vi "PH_Beckhoff-16BB.write Chiller to PSDB.vi"(0 "i ref in":refnum<vi>, 5 "error IO":errorcluster) -> (14 "i ref out":refnum<vi>, 19 "error out":errorcluster)   [LabVIEW 2014, in "PH_Beckhoff-16BB.lvlib"]
doc: "This VI writes the chiller data to the PHELIX shot data base."
uses:
  PH_Beckhoff-16BB.lvlib
  PH_StatusHandler/PH_StatusHandler.Status.ctl
  PH_PSDBWriter/PH_PSDBWriter.Data Status.ctl
  PH_Beckhoff/PH_Beckhoff.lvlib
  CSCore/CSSystem/CSSystemLib/CSSystemLib.lvlib
  PH_PSDBWriter/PH_PSDBWriter.lvlib
  PH_Common/PH_Common.lvlib
  PH_StatusHandler/PH_StatusHandler.lvlib
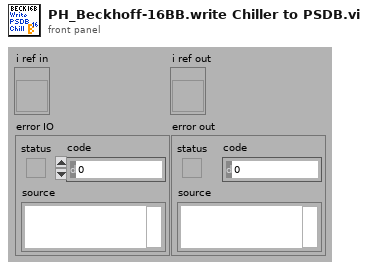
[diagram p1: front panel]
types:
  T1 = typedef "PH_Beckhoff.lvlib/PH_Beckhoff.i attribute.ctl" = cluster{"GUI Refs":T2, "operation?":bool, "Default Prdc Interval":i32, "Connection":T3, "AMS Net ID":T4, "Klemmencluster: # of":T5, "Values":T6, "IP":string, "Description":string, "configured?":bool, "Change Manager":cluster{"Detemination wanted?":bool, "Values changed at":cluster{"Sonderklemmen Inputs":i32[], "Analog Inputs":i32[], "Analog Outputs":i32[], "Digital Inputs":i32[], "Digital Outputs":i32[]}}, "Difference to handle an analog input as change":u32}
  T2 = typedef "PH_Beckhoff.lvlib/PH_Beckhoff.GUI Refs.ctl" = cluster{"ADS Error":refnum<vi>, "Values":refnum<vi>, "configured?":refnum<vi>, "Connection":refnum<vi>, "IP":refnum<vi>, "Prdc Int [ms]":refnum<vi>}
  T3 = typedef "PH_Beckhoff.lvlib/PH_Beckhoff.Connectivity.ctl" = cluster{"DLL?":bool, "Port?":bool, "Client?":bool, "Ping?":bool, "unsuccessful Pings":u32}
  T4 = typedef "Beckhoff - Driver np.lvlib/Beckhoff Access.ctl" = cluster{"DLL path":path, "AMS Net ID":cluster{"1st # of IP":u8, "2nd # of IP":u8, "3rd # of IP":u8, "4th # of IP":u8, "In Port":u8, "Out Port":u8}}
  T5 = typedef "Beckhoff - Driver np.lvlib/Klemmendeclarer.ctl" = cluster{"Offset due to Sonderklemms":u32, "analog Inputs":u32, "analog Outputs":u32, "digital Input Bits":u32, "digital Output Bits":u32}
  T6 = typedef "PH_Beckhoff.lvlib/PH_Beckhoff.Values.ctl" = cluster{"Sonderklemmen Inputs":T7, "Analog Inputs":T8, "Analog Outputs":T10, "Digital Inputs":T11, "Digital Outputs":T12}
  T7 = typedef "PH_Beckhoff.lvlib/PH_Beckhoff.Sonderklemmen Inputs.ctl" = cluster{"Total Length":u32, "Name":string, "Value":u64, "Quality":bool, "Service ID":i32, "Offset":u32, "Length":u32}[]
  T8 = typedef "PH_Beckhoff.lvlib/PH_Beckhoff.Analog Inputs.ctl" = cluster{"Name":string, "Value":u32, "Quality":bool, "Service ID":i32, "Sca Type":T9}[]
  T9 = typedef "PH_Beckhoff.lvlib/PH_Beckhoff.Scaling Type.ctl" = enum16{"none", "0 ... 15 Bit -> 0 ... 5", "0 ... 15 Bit -> 0 ... 10", "0 ... 15 Bit -> 0 ... 25", "0 ... 15 Bit -> 4 ... 20", "0 ... 15 Bit -> 0 ... 1", "0 ... 15 Bit -> 0 ... 20000", "0 ... 15 Bit -> 0 ... 24000"}
  T10 = typedef "PH_Beckhoff.lvlib/PH_Beckhoff.Analog Outputs.ctl" = cluster{"Name":string, "Value":u32, "Quality":bool, "Wanted Value":u32, "Service ID":i32, "Sca Type":T9}[]
  T11 = typedef "PH_Beckhoff.lvlib/PH_Beckhoff.Digital Inputs.ctl" = cluster{"Name":string, "Value":bool, "Quality":bool, "Service ID":i32, "inverted?":bool}[]
  T12 = typedef "PH_Beckhoff.lvlib/PH_Beckhoff.Digital Outputs.ctl" = cluster{"Name":string, "Value":bool, "Quality":bool, "Wanted Value":bool, "Service ID":i32, "inverted?":bool}[]
  T13 = typedef "PH_Beckhoff-16BB.lvlib/PH_Beckhoff-16BB.i attribute.ctl" = cluster{"PA Chiller":cluster{"PSDB":cluster{"Status Service ID":i32, "Instance ID":i32, "Data Status":T14, "Ref Status":refnum<vi>, "Error Code":i32}, "Status":cluster{"GUI Ref":refnum<vi>, "Status Service ID":i32, "Status":T15}, "DIs":cluster{"Flow Control":cluster{"GUI Ref":refnum<vi>, "# in Data":i32}, "High-Temp":cluster{"GUI Ref":refnum<vi>, "# in Data":i32}, "Conductivity":cluster{"GUI Ref":refnum<vi>, "# in Data":i32}, "Niveau":cluster{"GUI Ref":refnum<vi>, "# in Data":i32}}, "PSDB Thread":cluster{"Ref":refnum<vi>, "Q-Ref":refnum<queue>}}, "PSDB":cluster{"Shot #":i32, "Subsystem":T16}, "Racktype":string, "PSDB Credentials":T17}
  T14 = typedef "PH_PSDBWriter.lvlib/PH_PSDBWriter.Data Status.ctl" = i16
  T15 = typedef "PH_StatusHandler.lvlib/PH_StatusHandler.Status.ctl" = i16
  T16 = typedef "PH_PSDBWriter.lvlib/PH_PSDBWriter.PHELIX-Subsystems.ctl" = i32
  T17 = typedef "PH_Common.lvlib/PH_Connection.PSDB Credentials.ctl" = cluster{"PW":string, "ID":string, "DS":string}
  T18 = typedef "PH_PSDBWriter.lvlib/PH_PSDBWriter.String dataset.ctl" = cluster{"name":string, "data":string, "unit":string}
  T19 = typedef "PH_PSDBWriter.lvlib/PH_PSDBWriter.PSDB Dataset.ctl" = cluster{"Version":i32, "2D data Input":T20[], "Boolean Input":T22[], "Image Input":T23[], "Numeric Input":T25[], "String Input":T18[]}
  T20 = typedef "PH_PSDBWriter.lvlib/PH_PSDBWriter.2D dataset.ctl" = cluster{"name":string, "data":dbl[][], "axis description":T21}
  T21 = typedef "PSDB.lvlib/PSDB_AxisDescription.ctl" = cluster{"x axis label":string, "y axis label":string, "x axis unit":string, "y axis unit":string}
  T22 = typedef "PH_PSDBWriter.lvlib/PH_PSDBWriter.Boolean dataset.ctl" = cluster{"name":string, "data":bool, "unit":string}
  T23 = typedef "PH_PSDBWriter.lvlib/PH_PSDBWriter.Image dataset.ctl" = cluster{"name":string, "data":T24, "unit":string}
  T24 = typedef "IMAQ Image.ctl" = refnum<image>
  T25 = typedef "PH_PSDBWriter.lvlib/PH_PSDBWriter.Numeric dataset.ctl" = cluster{"name":string, "data":dbl, "unit":string}
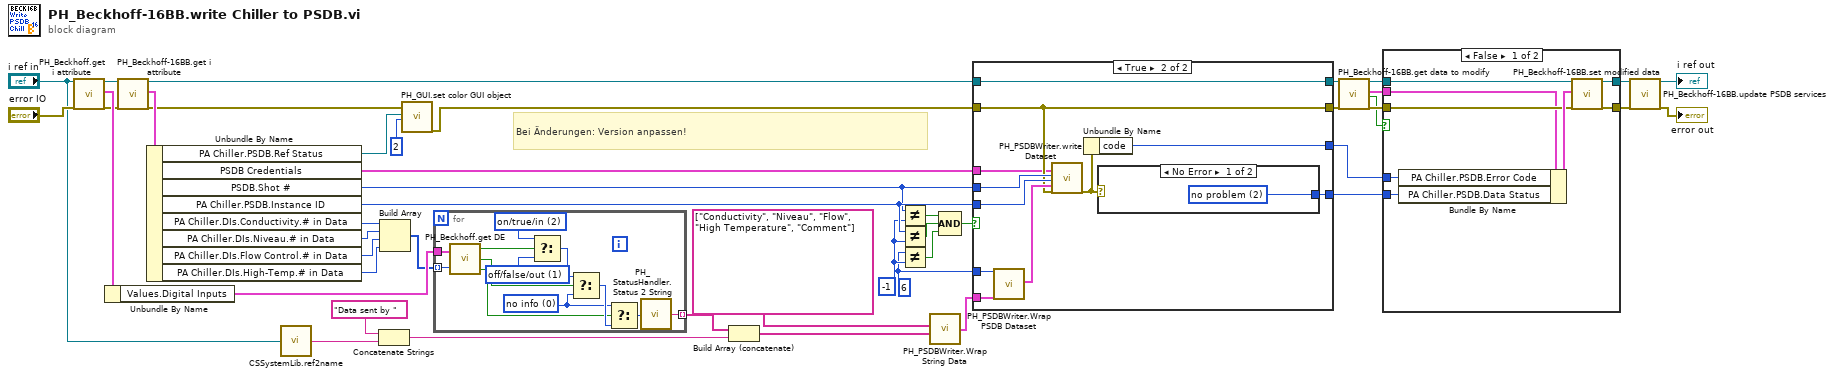
[diagram p0: block diagram]
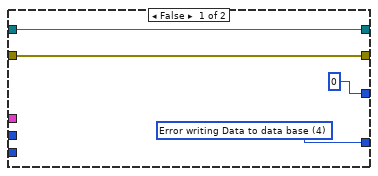
[diagram p3: hidden frame]
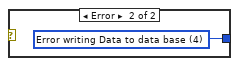
[diagram p4: hidden frame]
diagram:
  w34 = 6 ("Version")
  w40 = -1 ("y")
  # "Bei Änderungen: Version anpassen!"
  n1 = call "PH_Beckhoff.get i attribute.vi"("i ref in"="i ref in", "error in (no error)"="error IO") -> ("i ref out"=w12:refnum<vi>, "i attribute"=w23:T1, "error out"=w10:errorcluster)  [unwired: 15 in]
  n2 = Unbundle By Name(w23) -> ("Values.Digital Inputs"=w29:T11)
  n3 = call "PH_Beckhoff-16BB.get i attribute.vi"("i ref in"=w12, "error in (no error)"=w10) -> ("i ref out"=w11:refnum<vi>, "i attribute"=w9:T13, "error out"=w6:errorcluster)  [unwired: 15 in]
  n4 = Unbundle By Name(w9) -> ("PA Chiller.PSDB.Ref Status"=w8:refnum<vi>, "PSDB Credentials"=w1:T17, "PSDB.Shot #"=w42:i32, "PA Chiller.PSDB.Instance ID"=w43:i32, "PA Chiller.DIs.Conductivity.# in Data"=w33:i32, "PA Chiller.DIs.Niveau.# in Data"=w32:i32, "PA Chiller.DIs.Flow Control.# in Data"=w31:i32, "PA Chiller.DIs.High-Temp.# in Data"=w30:i32)
  n5 = call "CSSystemLib.ref2name.vi"("obj refnum"="i ref in") -> ("name"=w24:string)
  n6 = Concatenate Strings("Data sent by " ("string"), w24) -> (w25:string)
  n7 = Build Array(w33, w32, w31, w30) -> (w28:i32[])
  n8 = call "PH_GUI.set color GUI object.vi"("GUI object Ref"=w8, "State"=2, "error in (no error)"=w6) -> ("error out"=w5:errorcluster)  [unwired: 16 in]
  n9 = for {
    tunnel: [w51] -> w27 mode=indexing
    tunnel: w29 -> [w47]
    tunnel: w28 -> [w46] mode=indexing
    w53 = T15 1 items=["no info", "off/false/out", "on/true/in", "Failure", "Alarm", "Status 1", "Status 2", "Status 3"] ("State Temp not 2 low")
    w54 = T15 2 items=["no info", "off/false/out", "on/true/in", "Failure", "Alarm", "Status 1", "Status 2", "Status 3"] ("State Temp not 2 low")
    w56 = T15 0 items=["no info", "off/false/out", "on/true/in", "Failure", "Alarm", "Status 1", "Status 2", "Status 3"] ("State Temp not 2 low")
    n10 = call "PH_Beckhoff.get DE.vi"("Digital Values"=w47, "index of element"=w46) -> ("Value"=w50:bool, "Quality"=w49:bool, "Tag not found"=w48:bool)
    n11 = Select(t=w54, s=w50, f=w53) -> (s? t:f=w55:T15)
    n12 = Select(t=w55, s=w49, f=w56) -> (s? t:f=w57:T15)
    n13 = Select(t=w56, s=w48, f=w57) -> (s? t:f=w52:T15)
    n14 = call "PH_StatusHandler.Status 2 String.vi"("Status"=w52) -> ("Status as string"=w51:string)
  }
  n15 = Build Array (concatenate)(w27, w25) -> (w4:string[])
  n16 = Not Equal?(x=w42, y=w40) -> (x != y?=w39:bool)
  n17 = Not Equal?(x=w43, y=w40) -> (x != y?=w38:bool)
  n18 = Not Equal?(x=w34, y=w40) -> (x != y?=w37:bool)
  n19 = call "PH_PSDBWriter.Wrap String Data.vi"("Data Array"=w4, "Name Array"=string[] ["Conductivity", "Niveau", "Flow", "High Temperature", "Comment"]) -> ("PSDB String Data Array"=w2:T18[])  [unwired: 2 in]
  n20 = Compound Arithmetic op=AND(w39, w38, w37) -> (w36:bool)
  n21 = case shown="True" w36 {
    tunnel: w5 -> [w59 w65]
    tunnel: w43 -> [_ w66]
    tunnel: w34 -> [_ w69]
    tunnel: [w61 w72] -> w41
    tunnel: w11 -> [w60 w71]
    tunnel: [w60 w71] -> w21
    tunnel: [w59 w65] -> w19
    tunnel: w42 -> [_ w67]
    tunnel: [0 ("code") w70] -> w35
    tunnel: w2 -> [_ w63]
    tunnel: w1 -> [_ w62]
    frame False {
      w61 = T14 4 items=["no info", "no Data collection", "no problem", "Error getting the instance ID", "Error writing Data to data base", "Error concerning the subsystem"] ("Data Status")
    }
    frame True {
      n22 = call "PH_PSDBWriter.Wrap PSDB Dataset.vi"("Version"=w69, "String Input"=w63) -> ("PSDB Dataset"=w68:T19)  [unwired: 17 in]
      n23 = call "PH_PSDBWriter.write Dataset.vi"("PSDB Credentials"=w62, "Shot #"=w67, "Instance ID"=w66, "Data to write to PSDB"=w68, "error in (no error)"=w65) -> ("error out"=w64:errorcluster)  [unwired: 14 in]
      n24 = Unbundle By Name(w64) -> ("code"=w70:i32)
      n25 = case shown="No Error" w64 {
        tunnel: [w73 w74] -> w72
        frame No Error {
          w73 = T14 2 items=["no info", "no Data collection", "no problem", "Error getting the instance ID", "Error writing Data to data base", "Error concerning the subsystem"] ("Data Status")
        }
        frame Error {
          w74 = T14 4 items=["no info", "no Data collection", "no problem", "Error getting the instance ID", "Error writing Data to data base", "Error concerning the subsystem"] ("Data Status")
        }
      }
    }
  }
  n26 = call "PH_Beckhoff-16BB.get data to modify.vi"("i ref in"=w21, "error in (no error)"=w19) -> ("i ref out"=w22:refnum<vi>, "i attribute"=w18:T13, "timed out"=w17:bool, "error out"=w20:errorcluster)  [unwired: 14 in]
  n27 = case shown="False" w17 {
    tunnel: [w82 w84] -> w16
    tunnel: [w81 w83] -> w15
    tunnel: w41 -> [w80 _]
    tunnel: w35 -> [w78 _]
    tunnel: w22 -> [w77 w84]
    tunnel: w20 -> [w76 w83]
    tunnel: w18 -> [w75 _]
    frame False {
      n28 = Bundle By Name(cluster=w75, "PA Chiller.PSDB.Error Code"=w78, "PA Chiller.PSDB.Data Status"=w80) -> (w79:T13)
      n29 = call "PH_Beckhoff-16BB.set modified data.vi"("i ref in"=w77, "i attribute"=w79, "error in (no error)"=w76) -> ("i ref out"=w82:refnum<vi>, "error out"=w81:errorcluster)  [unwired: 15 in]
    }
    frame True {
    }
  }
  n30 = call "PH_Beckhoff-16BB.update PSDB services.vi"("i ref in"=w16, "error in"=w15) -> ("i ref out"=→"i ref out":refnum<vi>, "error out"=→"error out":errorcluster)  [unwired: 16 in]
